vi "Start Stop Trial.vi"(8 "error in (no error)":errorcluster, 10 "Acquiring true?":bool, 11 "Lissajous Viewer in":refnum<class "Lissajous Viewer.lvclass">) -> (0 "error out":errorcluster, 3 "Lissajous Viewer out":refnum<class "Lissajous Viewer.lvclass">)   [LabVIEW 2020, in "Lissajous Viewer.lvlib" / "Lissajous Viewer.lvclass"]
uses:
  Lissajous Viewer.lvclass
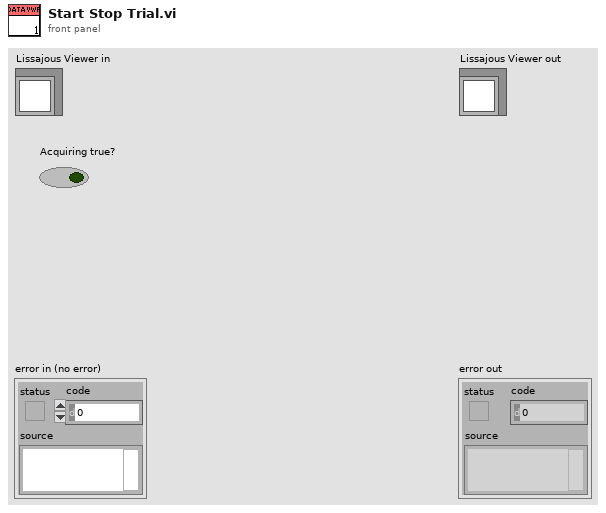
[diagram p1: front panel]
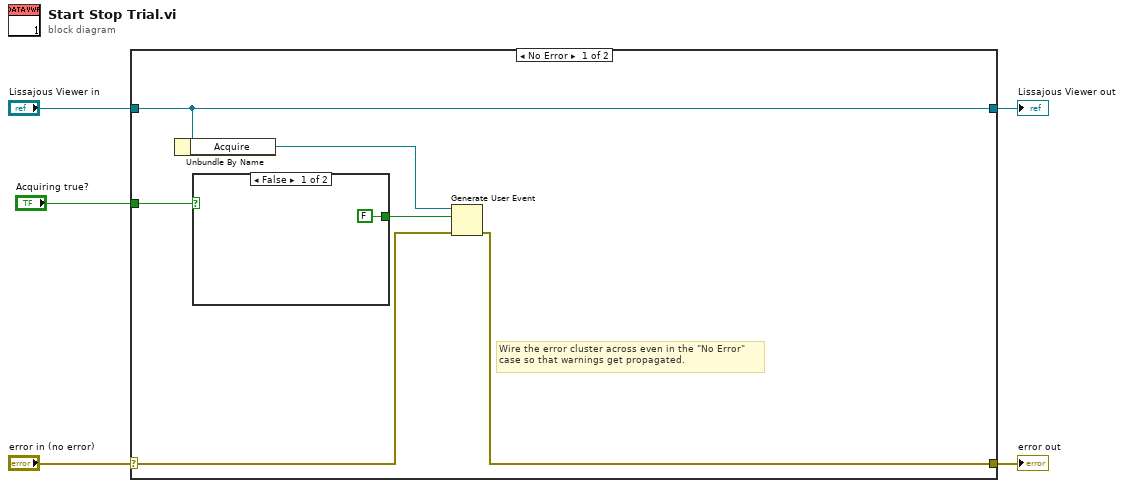
[diagram p0: block diagram]
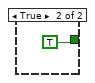
[diagram p2: hidden frame]
diagram:
  n1 = case shown="No Error" "error in (no error)" {
    selector: "error in (no error)" -> [w8 w15]
    tunnel: [w7 w15] -> w4
    tunnel: [w11 w14] -> w2
    tunnel: "Lissajous Viewer in" -> [w11 w14]
    tunnel: "Acquiring true?" -> [w10 _]
    frame No Error {
      # "Wire the error cluster across even in the \"No Error\"\ncase so that warnings get propagated."
      n2 = Unbundle By Name(w11) -> ("Acquire"=w9:refnum<user-event>)
      n3 = case shown="False" w10 {
        tunnel: [FALSE TRUE] -> w6
        frame False {
        }
        frame True {
        }
      }
      n4 = Generate User Event(user event=w9, event data cluster=w6, error in=w8) -> (error out=w7:errorcluster)  [unwired: 1 in, 1 out]
    }
    frame Error {
    }
  }
  "error out" <- w4
  "Lissajous Viewer out" <- w2
